vi "WPI_AccelerometerInfoString.vi"(11 "AccelerometerDevRef":T1 {"Device Address" format="%.0x"; "Accel Range" items=["+/- 2 g", "+/- 4 g", "+/- 8 g", "+/- 16 g"]}) -> (3 "String":string)   [LabVIEW 2017]
uses:
  <vilib>/Rock Robotics/WPI/Accelerometer/WPI_AccelerometerDevRef.ctl
  <vilib>/Rock Robotics/WPI/Accelerometer/WPI_AccelerometerScaling.ctl
  <vilib>/Rock Robotics/WPI/Accelerometer/WPI_AccelerometerAnalogChannels.ctl
  <vilib>/Rock Robotics/SystemInterfaces/AI/FPGA_AIChannel.ctl
  <vilib>/Rock Robotics/SystemInterfaces/i2clib/i2c_bus.ctl
  <vilib>/Rock Robotics/SystemInterfaces/spilib/spi_bus.ctl
  <vilib>/Rock Robotics/WPI/Accelerometer/ADXL345 Range.ctl
  <vilib>/Rock Robotics/WPI/Accelerometer/WPI_AccelerometerADXL345 Axes.ctl
panel:
  # "ADXL"
  # "Analog"
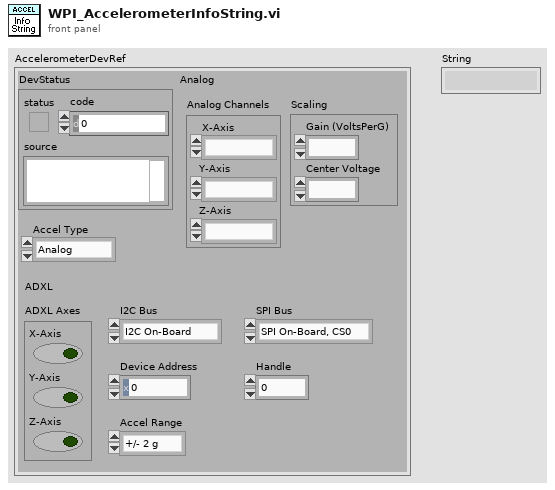
[diagram p1: front panel]
types:
  T1 = typedef "WPI_AccelerometerDevRef.ctl" = cluster{"DevStatus":errorcluster, "Scaling":T2, "Analog Channels":T3, "I2C Bus":T5, "SPI Bus":T6, "Accel Range":T7, "ADXL Axes":T8, "Handle":i32, "Device Address":u8, "Accel Type":enum16{"Analog", "ADXL345 I2C", "ADXL345 SPI", "Internal", "ADXL362 SPI"}}
  T2 = typedef "WPI_AccelerometerScaling.ctl" = cluster{"Gain (VoltsPerG)":dbl, "Center Voltage":dbl}
  T3 = typedef "WPI_AccelerometerAnalogChannels.ctl" = cluster{"X-Axis":T4, "Y-Axis":T4, "Z-Axis":T4}
  T4 = typedef "FPGA_AIChannel.ctl" = enum8{"AI 0", "AI 1", "AI 2", "AI 3", "AI MXP 0", "AI MXP 1", "AI MXP 2", "AI MXP 3", "Invalid"}
  T5 = typedef "i2c_bus.ctl" = enum16{"I2C On-Board", "I2C MXP", "Invalid"}
  T6 = typedef "spi_bus.ctl" = enum16{"SPI On-Board, CS0", "SPI On-Board, CS1", "SPI On-Board, CS2", "SPI On-Board, CS3", "SPI MXP", "Invalid"}
  T7 = typedef "ADXL345 Range.ctl" = u8
  T8 = typedef "WPI_AccelerometerADXL345 Axes.ctl" = cluster{"X-Axis":bool, "Y-Axis":bool, "Z-Axis":bool}
  T9 = enum16{"Analog", "ADXL345 I2C", "ADXL345 SPI", "Internal", "ADXL362 SPI"}
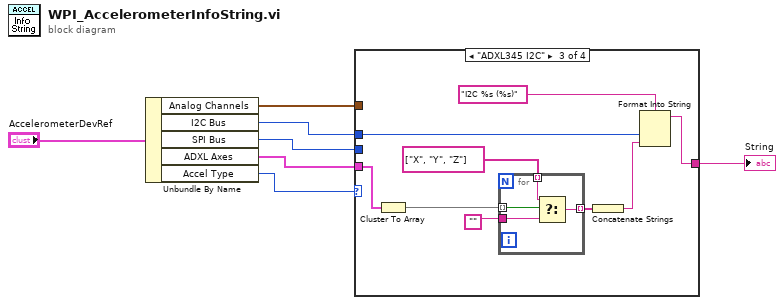
[diagram p0: block diagram]
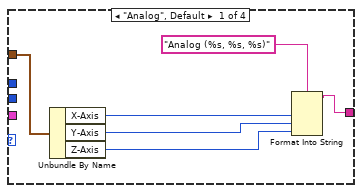
[diagram p2: hidden frame]
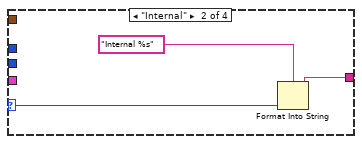
[diagram p3: hidden frame]
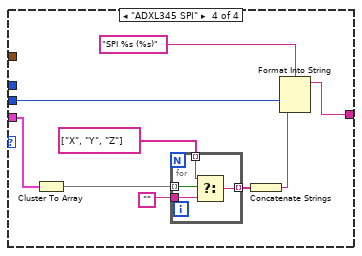
[diagram p4: hidden frame]
diagram:
  n1 = Unbundle By Name("AccelerometerDevRef") -> ("Analog Channels"=w5:T3, "I2C Bus"=w3:T5, "SPI Bus"=w1:T6, "ADXL Axes"=w2:T8, "Accel Type"=w4:T9)
  n2 = case shown="\"ADXL345 I2C\"" w4 {
    selector: w4 -> [_ w14 _ _]
    tunnel: [w8 w15 w17 w37] -> w7
    tunnel: w5 -> [w13 _ _ _]
    tunnel: w3 -> [_ _ w24 _]
    tunnel: w2 -> [_ _ w23 w31]
    tunnel: w1 -> [_ _ _ w36]
    frame "Analog", Default {
      n3 = Unbundle By Name(w13) -> ("X-Axis"=w11:T4, "Y-Axis"=w10:T4, "Z-Axis"=w9:T4)
      n4 = Format Into String(format string="Analog (%s, %s, %s)", w11, w10, w9) -> (resulting string=w8:string)  [unwired: 2 in, 1 out]
    }
    frame "Internal" {
      n5 = Format Into String(format string="Internal %s", w14) -> (resulting string=w15:string)  [unwired: 2 in, 1 out]
    }
    frame "ADXL345 I2C" {
      n6 = Cluster To Array(cluster=w23) -> (array=w22:bool[])
      n7 = for {
        tunnel: w22 -> [w29] mode=indexing
        tunnel: "" -> [w28]
        tunnel: string[] ["X", "Y", "Z"] -> [w27] mode=indexing
        tunnel: [w26] -> w19 mode=indexing
        n8 = Select(t=w27, s=w29, f=w28) -> (s? t:f=w26:string)
      }
      n9 = Concatenate Strings(w19) -> (w18:string)
      n10 = Format Into String(format string="I2C %s (%s)", w24, w18) -> (resulting string=w17:string)  [unwired: 2 in, 1 out]
    }
    frame "ADXL345 SPI" {
      n11 = Cluster To Array(cluster=w31) -> (array=w35:bool[])
      n12 = for {
        tunnel: w35 -> [w42] mode=indexing
        tunnel: "" -> [w41]
        tunnel: string[] ["X", "Y", "Z"] -> [w40] mode=indexing
        tunnel: [w39] -> w32 mode=indexing
        n13 = Select(t=w40, s=w42, f=w41) -> (s? t:f=w39:string)
      }
      n14 = Concatenate Strings(w32) -> (w30:string)
      n15 = Format Into String(format string="SPI %s (%s)", w36, w30) -> (resulting string=w37:string)  [unwired: 2 in, 1 out]
    }
  }
  "String" <- w7
